vi "Run_Module.vi"(0 "VI_In":refnum<vi>, 11 "Error_In":errorcluster) -> (4 "VI_Out":refnum<vi>, 15 "Error_Out":errorcluster)   [LabVIEW 2023]
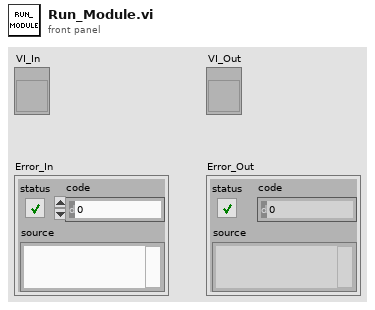
[diagram p1: front panel]
types:
  T1 = enum32{"Bad", "Idle", "Run top level", "Running"}
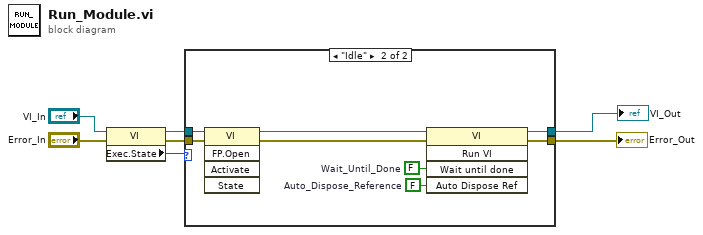
[diagram p0: block diagram]
diagram:
  n1 = property class="VI"(reference="VI_In", error in="Error_In") -> (reference out=w4:refnum<vi>, error out=w5:errorcluster, "Exec.State"=w7:T1)
  n2 = case shown="\"Idle\"" w7 {
    tunnel: [w9 w13] -> w1
    tunnel: [w8 w12] -> w2
    tunnel: w4 -> [w8 w11]
    tunnel: w5 -> [w9 w10]
    frame "Bad", Default {
    }
    frame "Idle" {
      w17 = FALSE  # Auto_Dispose_Reference
      w16 = FALSE  # Wait_Until_Done
      n3 = invoke on="Invoke Node" class="VI" method="FP.Open"(reference=w11, error in=w10) -> (reference out=w15:refnum<vi>, error out=w14:errorcluster)  [unwired: 3 in, 3 out]
      n4 = invoke on="Invoke Node" class="VI" method="Run VI"(reference=w15, error in=w14, "Wait until done"=w16, "Auto Dispose Ref"=w17) -> (reference out=w12:refnum<vi>, error out=w13:errorcluster)  [unwired: 1 in, 3 out]
    }
  }
  "VI_Out" <- w2
  "Error_Out" <- w1
